vi "_updateOnlineDisplay_LV.vi"(2 "show lifetime":bool, 3 "Raw Data":T1, 4 "mode":u16(ring) items=["init", "run"], 5 "rebinning":dbl=1.0 min=1.0 max=4000.0 step=1.0) -> (0 "lifetime histograms":cluster{dbl[], u32[]}[](array[cluster]), 1 "Timetraces":i32[][](array[numeric]))   [LabVIEW 2009]
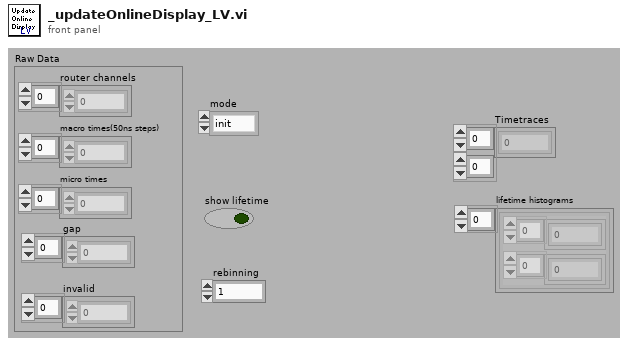
[diagram p1: front panel]
types:
  T1 = cluster{"router channels":u8[], "macro times(50ns steps)":u32[], "micro times":u16[], "gap":u32[], "invalid":u32[]}
  T2 = typedef "FIFOSettings.ctt" = cluster{"Measurement":cluster{"Binning (ms)":sgl, "External Trigger Condition":u16, "Stop Condition:":u16, "Stop Count":dbl, "Buffer Size (Photons)":u32, "No of Channels":u16, "Ext Latch Delay":i16}, "ADC":cluster{"Binning (HH)":i16, "Dither Range":i16, "Count Increment":i16, "Mode":u16}, "SYNC":cluster{"SYNC ZC Level (mV)":sgl, "SYNC Freq Divider":u16, "SYNC Holdoff (ps)":sgl, "SYNC Threshold (mV)":sgl}, "TAC":cluster{"TAC Range (ns)":sgl, "TAC Gain":i16, "TAC Offset (%)":sgl, "TAC Limit Low (%)":sgl, "TAC Limit High (%)":sgl}, "Ch 2":cluster{"Ch2 ZC Level (mV)":sgl, "Ch2 Holdoff (ps)":sgl, "Ch2 Threshold (mV)":sgl}, "Ch 3":cluster{"Ch3 ZC Level (mV)":sgl, "Ch3 Holdoff (ps)":sgl, "Ch3 Threshold (mV)":sgl}, "Ch 4":cluster{"Ch4 ZC Level (mV)":sgl, "Ch4 Holdoff (ps)":sgl, "Ch4 Threshold (mV)":sgl}, "Ch1":cluster{"Ch1 ZC Level (mV)":sgl, "Ch1 Holdoff (ps)":sgl, "Ch1 Threshold (mV)":sgl}}
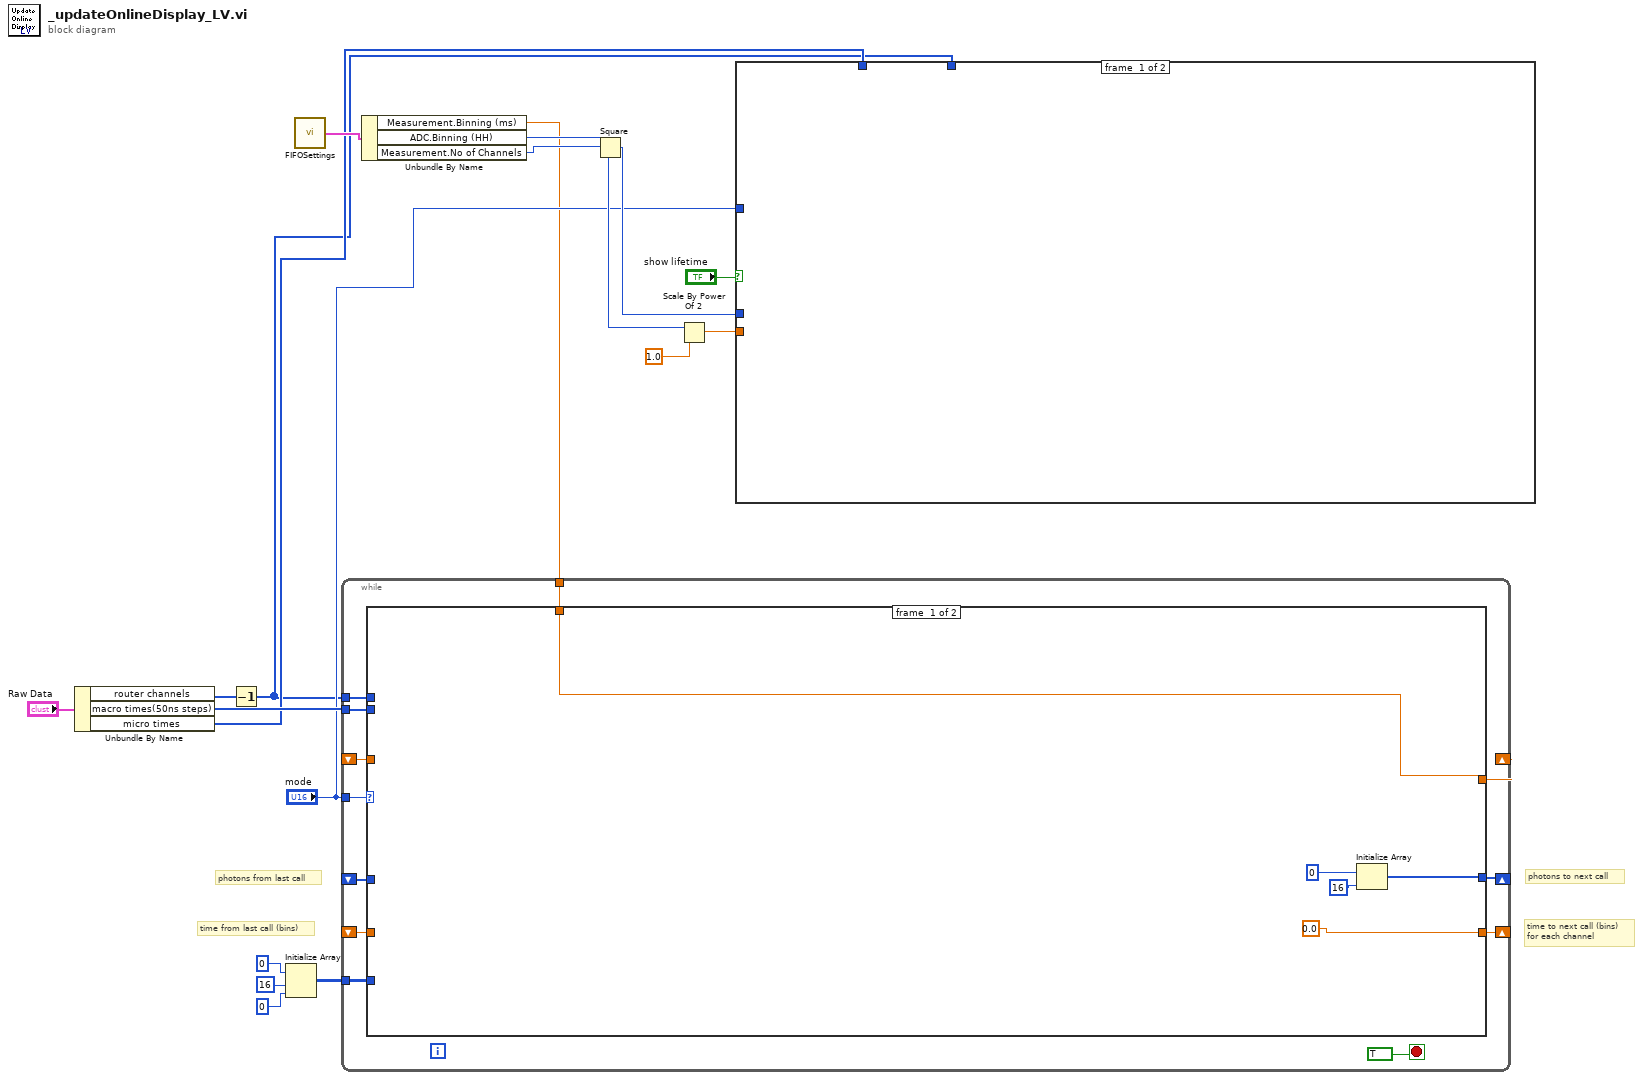
[diagram p0: block diagram]
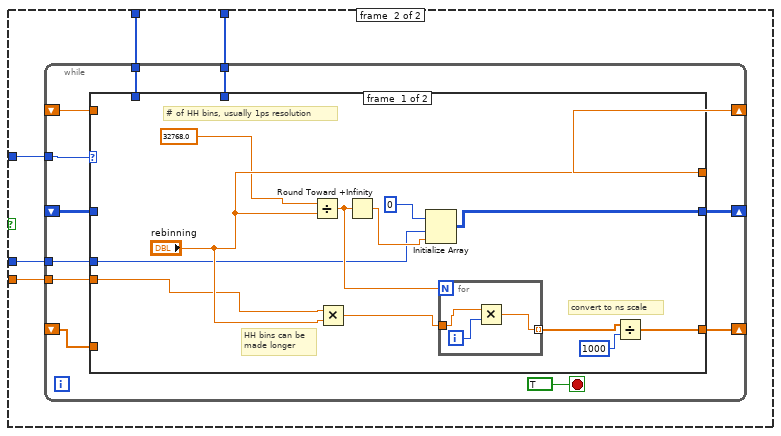
[diagram p2: hidden frame]
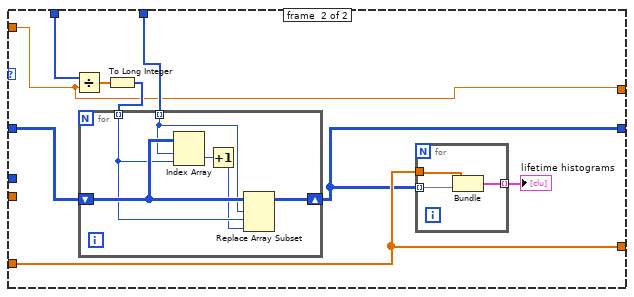
[diagram p3: hidden frame]
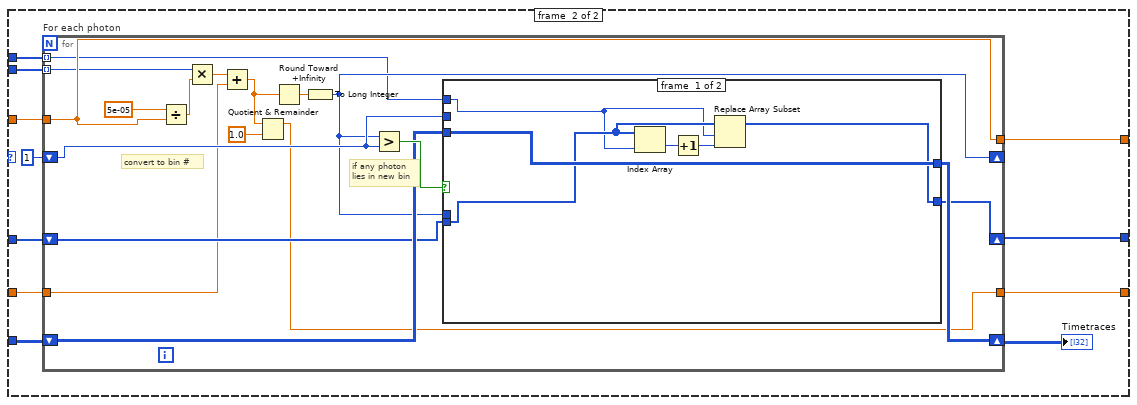
[diagram p4: hidden frame]
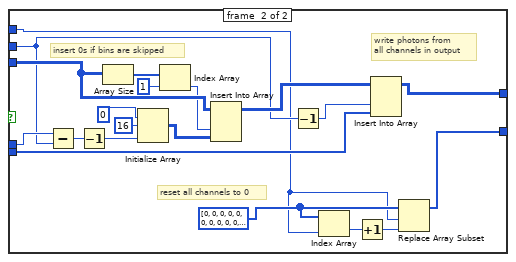
[diagram p5: hidden frame]
diagram:
  # "time to next call (bins)\nfor each channel"
  # "time from last call (bins)"
  # "photons to next call"
  # "photons from last call"
  n1 = Unbundle By Name("Raw Data") -> ("router channels"=w2:u8[], "macro times(50ns steps)"=w13:u32[], "micro times"=w4:u16[])
  n2 = Decrement(x=w2) -> (x-1=w1:u8[])
  n3 = Initialize Array(0 ("element"), 16 ("dimension size"), 0 ("dimension size")) -> (w15:i32[][])
  n4 = call "FIFOSettings.vi"() -> ("FIFO Settings(out)"=w12:T2)  [unwired: 2 in]
  n5 = Unbundle By Name(w12) -> ("Measurement.Binning (ms)"=w3:sgl, "ADC.Binning (HH)"=w10:i16, "Measurement.No of Channels"=w9:u16)
  n6 = while {
    shift-right: [w30] -> _
    shift-left: _ -> [w27]
    shift-right: [w29] -> _
    shift-left: _ -> [w28]
    shift-right: [w25] -> _
    shift-left: _ -> [w24]
    tunnel: "mode" -> [w23]
    tunnel: w13 -> [w22]
    tunnel: w1 -> [w21]
    tunnel: w15 -> [w20]
    tunnel: w3 -> [w19]
    stop <- TRUE stop-if-true
    n7 = case shown="1" w23 {
      tunnel: [w33 w46] -> w30
      tunnel: [0.0 w45] -> w29
      tunnel: w28 -> [_ w44]
      tunnel: w27 -> [_ w39]
      tunnel: [w31 w43] -> w25
      tunnel: w24 -> [_ w42]
      tunnel: w22 -> [_ w41]
      tunnel: w21 -> [_ w40]
      tunnel: w20 -> [_ w38]
      tunnel: w19 -> [w31 _]
      frame #0 {
        n8 = Initialize Array(0, 16 ("dimension size")) -> (w33:i32[])
      }
      frame #1 {
        n9 = for "For each photon" {
          tunnel: [w64] -> w43
          tunnel: w42 -> [w64]
          shift-right: [w49] -> w46
          shift-left: w39 -> [w51]
          tunnel: w41 -> [w59] mode=indexing
          tunnel: w40 -> [w50] mode=indexing
          shift-right: [w54] -> w36
          shift-left: w38 -> [w55]
          shift-right: [w52] -> _
          shift-left: 1 -> [w53]
          tunnel: w44 -> [w47]
          tunnel: [w48] -> w45
          # "if any photon\nlies in new bin"
          # "convert to bin #"
          n10 = Divide(x=5e-05 ("y"), y=w64) -> (x/y=w62:dbl)
          n11 = Multiply(x=w59, y=w62) -> (x*y=w61:dbl)
          n12 = Add(x=w61, y=w47) -> (x+y=w57:dbl)
          n13 = Quotient & Remainder(x=w57, y=1.0) -> (x-y*floor(x/y)=w48:dbl)  [unwired: 1 out]
          n14 = Round Toward +Infinity(x=w57) -> (ceil(x): smallest int >= x=w58:dbl)
          n15 = To Long Integer(number=w58) -> (32bit integer=w52:i32)
          n16 = Greater?(x=w52, y=w53) -> (0:w56:bool)
          n17 = case shown="True" w56 {
            tunnel: w51 -> [w67 w88]
            tunnel: w55 -> [w70 w78]
            tunnel: [w70 w89] -> w54
            tunnel: w50 -> [w66 w71]
            tunnel: w53 -> [_ w73]
            tunnel: [w65 w72] -> w49
            tunnel: w52 -> [_ w87]
            frame #0 {
              n18 = Index Array(array=w67, index=w66) -> (element=w69:i32)
              n19 = Increment(x=w69) -> (x+1=w68:i32)
              n20 = Replace Array Subset(array=w67, new element=w68, index=w66) -> (w65:i32[])
            }
            frame #1 {
              w74 = i32[] [0, 0, 0, 0, 0, 0, 0, 0, 0, 0, 0, 0, 0, 0, 0, 0] ("initialized array")
              # "reset all channels to 0"
              # "write photons from\nall channels in output"
              # "insert 0s if bins are skipped"
              n21 = Subtract(x=w87, y=w73) -> (x-y=w86:i32)
              n22 = Decrement(x=w86) -> (x-1=w85:i32)
              n23 = Array Size(array=w78) -> (size(s)=w80:i32[])
              n24 = Initialize Array(0 ("disabled index (col)"), 16 ("dimension size"), w85) -> (w82:i32[][])
              n25 = Index Array(array=w80, index=1) -> (element=w77:i32)
              n26 = Insert Into Array(array=w78, index (col)=w77, new element=w82) -> (w81:i32[][])  [unwired: 1 in]
              n27 = Decrement(x=w73) -> (x-1=w90:i32)
              n28 = Index Array(array=w74, index=w71) -> (element=w76:i32)
              n29 = Increment(x=w76) -> (x+1=w75:i32)
              n30 = Insert Into Array(array=w81, index (col)=w90, new element=w88) -> (w89:i32[][])  [unwired: 1 in]
              n31 = Replace Array Subset(array=w74, new element=w75, index=w71) -> (w72:i32[])
            }
          }
        }
        "Timetraces" <- w36
      }
    }
  }
  n32 = Square(x=w9) -> (x^2=w7:u16)
  n33 = Scale By Power Of 2(n=w10, x=1.0) -> (x*2^n=w8:dbl)
  n34 = case shown="True" "show lifetime" {
    tunnel: w1 -> [_ w95]
    tunnel: w4 -> [_ w94]
    tunnel: "mode" -> [_ w93]
    tunnel: w8 -> [_ w92]
    tunnel: w7 -> [_ w91]
    frame #0 {
    }
    frame #1 {
      n35 = while {
        tunnel: w95 -> [w106]
        shift-right: [w104] -> _
        shift-left: _ -> [w107]
        tunnel: w94 -> [w103]
        shift-right: [w101] -> _
        shift-left: _ -> [w102]
        shift-right: [w100] -> _
        shift-left: _ -> [w99]
        tunnel: w92 -> [w98]
        tunnel: w91 -> [w97]
        tunnel: w93 -> [w96]
        stop <- TRUE stop-if-true
        n36 = case shown="0, Default" w96 {
          tunnel: w107 -> [_ w131]
          tunnel: w106 -> [_ w130]
          tunnel: [w117 w123] -> w104
          tunnel: w103 -> [_ w128]
          tunnel: w102 -> [_ w126]
          tunnel: ["rebinning" w126] -> w101
          tunnel: [w110 w124] -> w100
          tunnel: w99 -> [_ w124]
          tunnel: w98 -> [w109 _]
          tunnel: w97 -> [w108 _]
          frame #0 {
            # "convert to ns scale"
            # "HH bins can be\nmade longer"
            # "# of HH bins, usually 1ps resolution"
            n37 = Divide(x=32768.0 ("channel count"), y="rebinning") -> (x/y=w115:dbl)
            n38 = Multiply(x=w109, y="rebinning") -> (x*y=w113:dbl)
            n39 = Round Toward +Infinity(x=w115) -> (ceil(x): smallest int >= x=w119:dbl)
            n40 = Initialize Array(u32 0 ("element"), w108, w119) -> (w117:u32[][])
            n41 = for {
              N: w115 -> [_]
              tunnel: [w121] -> w112 mode=indexing
              tunnel: w113 -> [w120]
              i -> [w122]
              n42 = Multiply(x=w120, y=w122) -> (x*y=w121:dbl)
            }
            n43 = Divide(x=w112, y=u32 1000 ("element")) -> (x/y=w110:dbl[])
          }
          frame #1 {
            n44 = Divide(x=w128, y=w126) -> (x/y=w129:dbl[])
            n45 = To Long Integer(number=w129) -> (32bit integer=w127:i32[])
            n46 = for {
              tunnel: w127 -> [w138] mode=indexing
              shift-right: [w137] -> w123
              shift-left: w131 -> [w140]
              tunnel: w130 -> [w139] mode=indexing
              n47 = Index Array(array=w140, index (row)=w139, index (col)=w138) -> (element=w136:u32)
              n48 = Increment(x=w136) -> (x+1=w135:u32)
              n49 = Replace Array Subset(array=w140, new element=w135, index (row)=w139, index (col)=w138) -> (w137:u32[][])
            }
            n50 = for {
              tunnel: w123 -> [w134] mode=indexing
              tunnel: w124 -> [w133]
              tunnel: [w132] -> w125 mode=indexing
              n51 = Bundle(w133, w134) -> (w132:cluster{dbl[], u32[]})  [unwired: 1 in]
            }
            "lifetime histograms" <- w125
          }
        }
      }
    }
  }
